vi "XY Graph Delete Successive Plots.vi"(8 "Error In":errorcluster, 9 "Plot Indices":i32[](array[numeric]), 11 "XYGraph Ref":refnum<vi>) -> (0 "Error Out":errorcluster, 1 "Plot Names":string[](array[string]), 2 "Graph Caption":string, 3 "XYGraph Ref":refnum<vi>)   [LabVIEW 2019, in "XY Graph Add-Ons.lvlib"]
uses:
  XY Graph Add-Ons.lvlib
  Plot Update Steps.ctl
  XY Graph Plot Properties.ctl
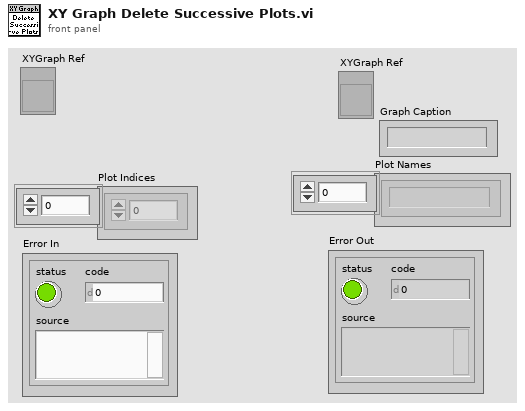
[diagram p1: front panel]
types:
  T1 = typedef "Plot Update Steps.ctl" = enum16{"Update Plot Styles", "Update Annotation List", "Update Cursor List", "Update Plots", "Quit"}
  T2 = typedef "XY Graph Plot Properties.ctl" = cluster{"Plot Index":i32, "Plot.Bar Plot Style":u8, "Plot.DigitalLineStyle":u8, "Plot.TransitionLocation":u8, "Plot.Transition Type":u8, "Plot.Fill To":i16, "Plot.Fill/Pt. Color":u32, "Plot.Label Format":u8, "Plot.Line Style":u8, "Plot.Line Width":u8, "Plot.Plot Color":u32, "Plot.Plot Interpolation":u8, "Plot.Plot Name":string, "Plot.Point Style":u8, "Plot.Visible?":bool, "Plot.XScaleIdx":u32, "Plot.YScaleIdx":u32, "Plot.Anti-aliased":bool}
  T3 = typedef "LVAnnotationListTypeDef.ctl" = cluster{"Name":string, "Color":u32, "Style":u8, "Point Style":u8, "Name Visible":bool, "Allow Drag":bool, "Annotation Mode":u32, "Plot":i32, "Index":i32, "Position":cluster{"X":dbl, "Y":dbl}, "X Scale":u32, "Y Scale":u32, "Show Arrow":bool, "Lock Name":bool, "Plot Area":i32, "Label Offset":cluster{"X":dbl, "Y":dbl}}[]
  T4 = typedef "LVCursorListTypeDef.ctl" = cluster{"Name":string, "Color":u32, "Style":u8, "Point Style":u8, "Name Visible":bool, "Allow Drag":bool, "Cursor Mode":u32, "Plot":i32, "Index":i32, "Position":cluster{"X":dbl, "Y":dbl}, "X Scale":u32, "Y Scale":u32, "Watch Plots":i32[], "Watch All Plots":bool, "Plot Area":i32, "Label Offset":cluster{"X":dbl, "Y":dbl}}[]
  T5 = typedef "XY Graph Add-Ons.lvlib/XY Graph Refnum.ctl" = refnum<vi>
  T6 = cluster{"Name":string, "Color":u32, "Style":u8, "Point Style":u8, "Name Visible":bool, "Allow Drag":bool, "Annotation Mode":u32, "Plot":i32, "Index":i32, "Position":cluster{"X":dbl, "Y":dbl}, "X Scale":u32, "Y Scale":u32, "Show Arrow":bool, "Lock Name":bool, "Plot Area":i32, "Label Offset":cluster{"X":dbl, "Y":dbl}}
  T7 = cluster{"Name":string, "Color":u32, "Style":u8, "Point Style":u8, "Name Visible":bool, "Allow Drag":bool, "Cursor Mode":u32, "Plot":i32, "Index":i32, "Position":cluster{"X":dbl, "Y":dbl}, "X Scale":u32, "Y Scale":u32, "Watch Plots":i32[], "Watch All Plots":bool, "Plot Area":i32, "Label Offset":cluster{"X":dbl, "Y":dbl}}
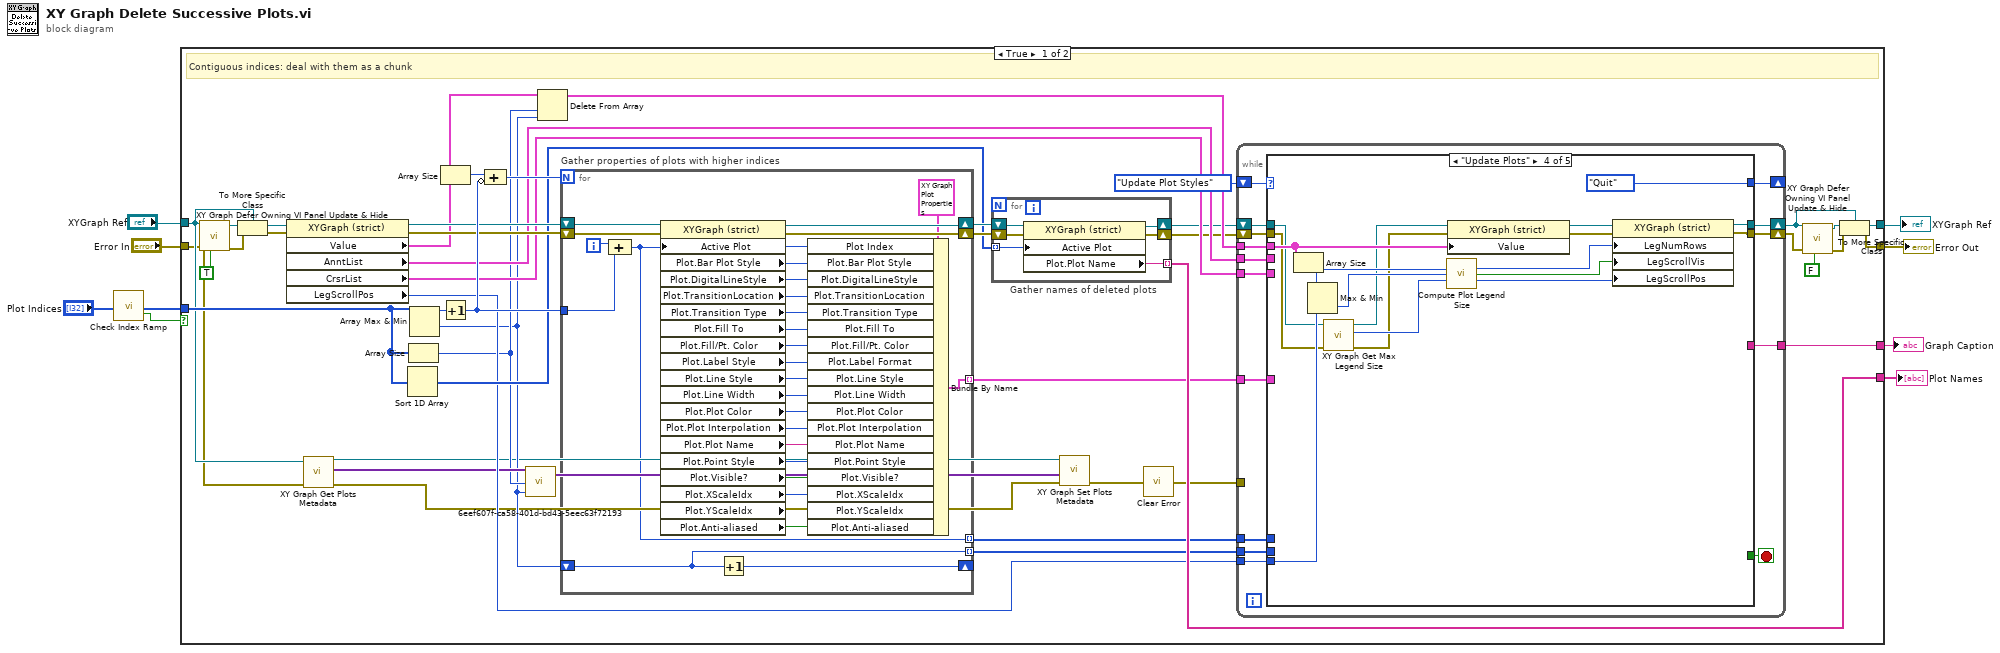
[diagram p0: block diagram]
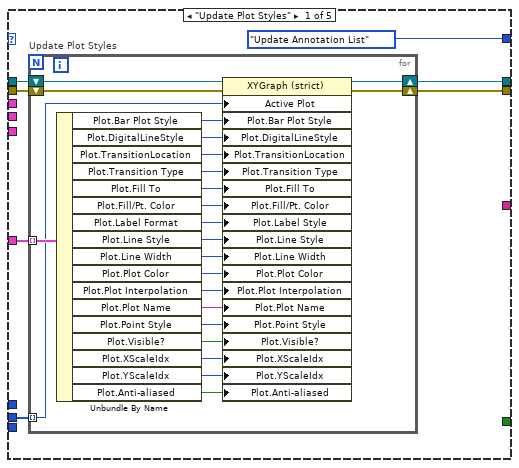
[diagram p2: hidden frame]
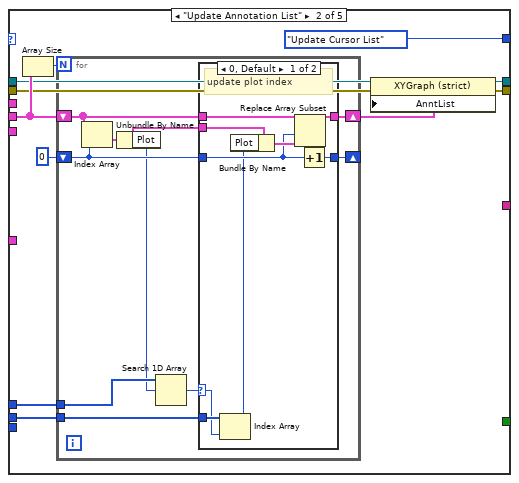
[diagram p3: hidden frame]
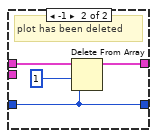
[diagram p4: hidden frame]
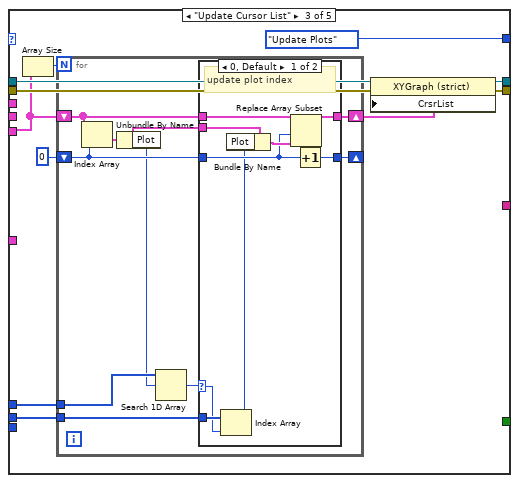
[diagram p5: hidden frame]
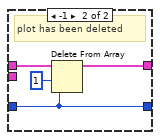
[diagram p6: hidden frame]
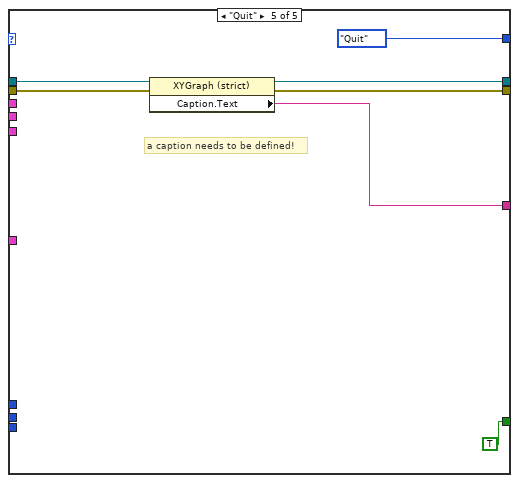
[diagram p7: hidden frame]
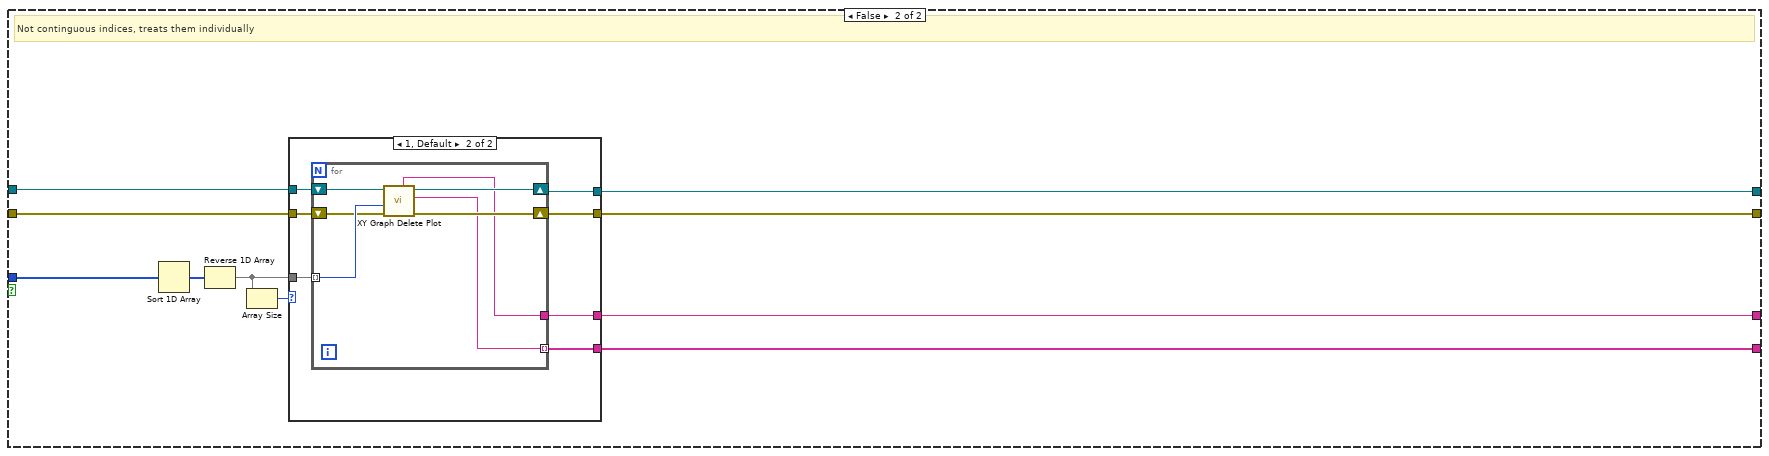
[diagram p8: hidden frame]
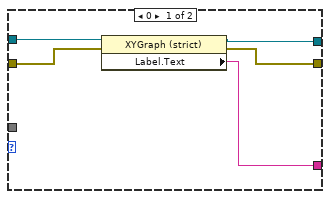
[diagram p9: hidden frame]
diagram:
  n1 = call "Check Index Ramp.vi"("Plot Indices"="Plot Indices") -> ("Plot Indices (dup)"=w1:i32[], "Contiguous?"=w2:bool)  [unwired: 16 in, 1 out]
  n2 = case shown="True" w2 {
    tunnel: "XYGraph Ref" -> [w19 w231]
    tunnel: [w23 w230] -> w8
    tunnel: "Error In" -> [w18 w229]
    tunnel: [w20 w228] -> w6
    tunnel: [w39 w227] -> w5
    tunnel: [w40 w226] -> w4
    tunnel: w1 -> [w46 w233]
    frame True {
      # "Contiguous indices: deal with them as a chunk"
      n3 = call "XY Graph Defer Owning VI Panel Update & Hide.vi"("Defer Owning Panel Update"=TRUE, "error in (no error)"=w18, "XY Graph Refnum in"=w19) -> ("error out"=w24:errorcluster, "XY Graph Refnum out"=w28:refnum<vi>)  [unwired: 7 in]
      n4 = To More Specific Class(target class=w19, reference=w28, error in=w24) -> (specific class reference=w26:refnum<vi>, error out=w25:errorcluster)
      n5 = property class="XYGraph (strict)"(reference=w26, error in=w25) -> (reference out=w49:refnum<vi>, error out=w48:errorcluster, "Value"=w47:cluster{dbl[], dbl[]}[], "AnntList"=w42:T3, "CrsrList"=w41:T4, "LegScrollPos"=w34:u32)
      n6 = call "XY Graph Get Plots Metadata.vi"("Error In"=w18, "XYGraph Refnum"=w19) -> ("Error Out"=w14:errorcluster, "Plots Metadata"=w17:variant[], "XYGraph Refnum"=w10:T5)  [unwired: 6 in, 1 out]
      n7 = Sort 1D Array(array=w46) -> (sorted array=w35:i32[])
      n8 = Array Size(array=w46) -> (size(s)=w16:i32)
      n9 = Array Max & Min(array=w46) -> (max value=w51:i32, min value=w15:i32)  [unwired: 2 out]
      n10 = Array Size(array=w47) -> (size(s)=w54:i32)
      n11 = Increment(x=w51) -> (x+1=w50:i32)
      n12 = Compound Arithmetic op=ADD(w54, invert w50) -> (w52:i32)
      n13 = call "6eef607f-ca58-401d-bd43-5eec63f72193.vi"("index (last elem)"=w15, "length (1)"=w16, "Array"=w17) -> ("array w/ subset deleted"=w11:variant[])  [unwired: 1 out]
      n14 = Delete From Array(array=w47, length=w16, index=w15) -> (array with subset deleted=w45:cluster{dbl[], dbl[]}[])  [unwired: 1 out]
      n15 = for "Gather properties of plots with higher indices" {
        N: w52 -> [_]
        shift-right: [w213] -> w43
        shift-left: w48 -> [w214]
        shift-right: [w215] -> w44
        shift-left: w49 -> [w217]
        tunnel: w50 -> [w195]
        shift-right: [w194] -> _
        shift-left: w15 -> [w193]
        tunnel: [w193] -> w38 mode=indexing
        tunnel: [w192] -> w37 mode=indexing
        tunnel: [w191] -> w36 mode=indexing
        i -> [w216]
        n16 = Compound Arithmetic op=ADD(w216, w195) -> (w191:i32)
        n17 = property class="XYGraph (strict)"(reference=w217, error in=w214, "Active Plot"=w191) -> (reference out=w215:refnum<vi>, error out=w213:errorcluster, "Plot.Bar Plot Style"=w212:u8, "Plot.DigitalLineStyle"=w211:u8, "Plot.TransitionLocation"=w210:u8, "Plot.Transition Type"=w209:u8, "Plot.Fill To"=w208:i16, "Plot.Fill/Pt. Color"=w207:u32, "Plot.Label Style"=w206:u8, "Plot.Line Style"=w205:u8, "Plot.Line Width"=w204:u8, "Plot.Plot Color"=w203:u32, "Plot.Plot Interpolation"=w202:u8, "Plot.Plot Name"=w201:string, "Plot.Point Style"=w200:u8, "Plot.Visible?"=w199:bool, "Plot.XScaleIdx"=w198:u32, "Plot.YScaleIdx"=w197:u32, "Plot.Anti-aliased"=w190:bool)
        n18 = Increment(x=w193) -> (x+1=w194:i32)
        n19 = Bundle By Name(cluster=T2 {"Plot Index"=0, "Plot.Bar Plot Style"=0, "Plot.DigitalLineStyle"=0, "Plot.TransitionLocation"=0, "Plot.Transition Type"=0, "Plot.Fill To"=0, "Plot.Fill/Pt. Color"=0, "Plot.Label Format"=0, "Plot.Line Style"=0, "Plot.Line Width"=0, "Plot.Plot Color"=0, "Plot.Plot Interpolation"=0, "Plot.Plot Name"="", "Plot.Point Style"=0, "Plot.Visible?"=FALSE, "Plot.XScaleIdx"=0, "Plot.YScaleIdx"=0, "Plot.Anti-aliased"=FALSE}, "Plot Index"=w191, "Plot.Bar Plot Style"=w212, "Plot.DigitalLineStyle"=w211, "Plot.TransitionLocation"=w210, "Plot.Transition Type"=w209, "Plot.Fill To"=w208, "Plot.Fill/Pt. Color"=w207, "Plot.Label Format"=w206, "Plot.Line Style"=w205, "Plot.Line Width"=w204, "Plot.Plot Color"=w203, "Plot.Plot Interpolation"=w202, "Plot.Plot Name"=w201, "Plot.Point Style"=w200, "Plot.Visible?"=w199, "Plot.XScaleIdx"=w198, "Plot.YScaleIdx"=w197, "Plot.Anti-aliased"=w190) -> (w192:T2)
      }
      n20 = for "Gather names of deleted plots" {
        shift-right: [w220] -> w32
        shift-left: w43 -> [w221]
        shift-right: [w222] -> w33
        shift-left: w44 -> [w223]
        tunnel: w35 -> [w219] mode=indexing
        tunnel: [w218] -> w40 mode=indexing
        n21 = property class="XYGraph (strict)"(reference=w223, error in=w221, "Active Plot"=w219) -> (reference out=w222:refnum<vi>, error out=w220:errorcluster, "Plot.Plot Name"=w218:string)
      }
      n22 = call "XY Graph Set Plots Metadata.vi"("error in (no error)"=w14, "Plots Metadata"=w11, "XY Graph Refnum"=w10) -> ("error out"=w13:errorcluster)  [unwired: 7 in, 1 out]
      n23 = call "Clear Error.vi"("Error In"=w13) -> ("no Error Out"=w12:errorcluster)  [unwired: 8 in]
      n24 = while {
        shift-right: [w64] -> _
        shift-left: Plot_Update_Steps."Update Plot Styles" -> [w66]
        shift-right: [w60] -> w31
        shift-left: w32 -> [w68]
        tunnel: w42 -> [w63]
        tunnel: w45 -> [w62]
        tunnel: w41 -> [w61]
        shift-right: [w67] -> w22
        shift-left: w33 -> [w69]
        tunnel: [w59] -> w39
        tunnel: w38 -> [w58]
        tunnel: w37 -> [w57]
        tunnel: w36 -> [w56]
        tunnel: w34 -> [w55]
        tunnel: w12 -> [_]
        stop <- w65 stop-if-true
        n25 = case shown="\"Update Plots\"" w66 {
          tunnel: w69 -> [w76 w106 w139 w168 w188]
          tunnel: w68 -> [w75 w104 w137 w169 w185]
          tunnel: [w74 w103 w136 w178 w184] -> w60
          tunnel: [w73 w105 w138 w179 w186] -> w67
          tunnel: w58 -> [w70 w101 w142 _ _]
          tunnel: [_ _ _ _ TRUE] -> w65
          tunnel: [Plot_Update_Steps."Update Annotation List" Plot_Update_Steps."Update Cursor List" Plot_Update_Steps."Update Plots" Plot_Update_Steps."Quit" Plot_Update_Steps."Quit"] -> w64
          tunnel: w63 -> [_ w109 _ _ _]
          tunnel: w62 -> [_ _ _ w181 _]
          tunnel: w61 -> [_ _ w134 _ _]
          tunnel: [_ _ _ _ w183] -> w59
          tunnel: w57 -> [w71 _ _ _ _]
          tunnel: w56 -> [_ w100 w133 _ _]
          tunnel: w55 -> [_ _ _ w175 _]
          frame "Update Plot Styles" {
            n26 = for "Update Plot Styles" {
              tunnel: w71 -> [w99] mode=indexing
              shift-right: [w95] -> w74
              shift-left: w75 -> [w96]
              shift-right: [w97] -> w73
              shift-left: w76 -> [w98]
              tunnel: w70 -> [w78] mode=indexing
              n27 = Unbundle By Name(w99) -> ("Plot.Bar Plot Style"=w94:u8, "Plot.DigitalLineStyle"=w93:u8, "Plot.TransitionLocation"=w92:u8, "Plot.Transition Type"=w91:u8, "Plot.Fill To"=w90:i16, "Plot.Fill/Pt. Color"=w89:u32, "Plot.Label Format"=w88:u8, "Plot.Line Style"=w87:u8, "Plot.Line Width"=w86:u8, "Plot.Plot Color"=w85:u32, "Plot.Plot Interpolation"=w84:u8, "Plot.Plot Name"=w83:string, "Plot.Point Style"=w82:u8, "Plot.Visible?"=w81:bool, "Plot.XScaleIdx"=w80:u32, "Plot.YScaleIdx"=w79:u32, "Plot.Anti-aliased"=w77:bool)
              n28 = property class="XYGraph (strict)"(reference=w98, error in=w96, "Active Plot"=w78, "Plot.Bar Plot Style"=w94, "Plot.DigitalLineStyle"=w93, "Plot.TransitionLocation"=w92, "Plot.Transition Type"=w91, "Plot.Fill To"=w90, "Plot.Fill/Pt. Color"=w89, "Plot.Label Style"=w88, "Plot.Line Style"=w87, "Plot.Line Width"=w86, "Plot.Plot Color"=w85, "Plot.Plot Interpolation"=w84, "Plot.Plot Name"=w83, "Plot.Point Style"=w82, "Plot.Visible?"=w81, "Plot.XScaleIdx"=w80, "Plot.YScaleIdx"=w79, "Plot.Anti-aliased"=w77) -> (reference out=w97:refnum<vi>, error out=w95:errorcluster)
            }
          }
          frame "Update Annotation List" {
            n29 = Array Size(array=w109) -> (size(s)=w108:i32)
            n30 = for {
              N: w108 -> [_]
              shift-right: [w116] -> w102
              shift-left: w109 -> [w118]
              shift-right: [w115] -> _
              shift-left: 0 -> [w117]
              tunnel: w101 -> [w111]
              tunnel: w100 -> [w114]
              n31 = Index Array(array=w118, index=w117) -> (element=w119:T6)
              n32 = Unbundle By Name(w119) -> ("Plot"=w113:i32)
              n33 = Search 1D Array(1D array=w114, element=w113) -> (index of element=w112:i32)  [unwired: 1 in]
              n34 = case shown="0, Default" w112 {
                selector: w112 -> [w121 _]
                tunnel: w119 -> [w128 _]
                tunnel: w118 -> [w126 w132]
                tunnel: w117 -> [w124 w129]
                tunnel: [w123 w130] -> w116
                tunnel: [w127 w129] -> w115
                tunnel: w111 -> [w122 _]
                frame 0, Default {
                  # "update plot index"
                  n35 = Index Array(array=w122, index=w121) -> (element=w120:i32)
                  n36 = Bundle By Name(cluster=w128, "Plot"=w120) -> (w125:T6)
                  n37 = Replace Array Subset(array=w126, new element=w125, index=w124) -> (w123:T3)
                  n38 = Increment(x=w124) -> (x+1=w127:i32)
                }
                frame -1 {
                  # "plot has been deleted"
                  n39 = Delete From Array(array=w132, length=1, index=w129) -> (array with subset deleted=w130:T3)  [unwired: 1 out]
                }
              }
            }
            n40 = property class="XYGraph (strict)"(reference=w106, error in=w104, "AnntList"=w102) -> (reference out=w105:refnum<vi>, error out=w103:errorcluster)
          }
          frame "Update Cursor List" {
            n41 = Array Size(array=w134) -> (size(s)=w141:i32)
            n42 = for {
              N: w141 -> [_]
              tunnel: w142 -> [w144]
              shift-right: [w149] -> w135
              shift-left: w134 -> [w151]
              shift-right: [w148] -> _
              shift-left: 0 -> [w150]
              tunnel: w133 -> [w147]
              n43 = Index Array(array=w151, index=w150) -> (element=w152:T7)
              n44 = Unbundle By Name(w152) -> ("Plot"=w146:i32)
              n45 = Search 1D Array(1D array=w147, element=w146) -> (index of element=w145:i32)  [unwired: 1 in]
              n46 = case shown="0, Default" w145 {
                selector: w145 -> [w154 _]
                tunnel: w152 -> [w161 _]
                tunnel: w151 -> [w159 w165]
                tunnel: w150 -> [w157 w162]
                tunnel: [w156 w163] -> w149
                tunnel: [w160 w162] -> w148
                tunnel: w144 -> [w155 _]
                frame 0, Default {
                  # "update plot index"
                  n47 = Index Array(array=w155, index=w154) -> (element=w153:i32)
                  n48 = Bundle By Name(cluster=w161, "Plot"=w153) -> (w158:T7)
                  n49 = Replace Array Subset(array=w159, new element=w158, index=w157) -> (w156:T4)
                  n50 = Increment(x=w157) -> (x+1=w160:i32)
                }
                frame -1 {
                  # "plot has been deleted"
                  n51 = Delete From Array(array=w165, length=1, index=w162) -> (array with subset deleted=w163:T4)  [unwired: 1 out]
                }
              }
            }
            n52 = property class="XYGraph (strict)"(reference=w139, error in=w137, "CrsrList"=w135) -> (reference out=w138:refnum<vi>, error out=w136:errorcluster)
          }
          frame "Update Plots" {
            n53 = Array Size(array=w181) -> (size(s)=w176:i32)
            n54 = Max & Min(x=w176, y=w175) -> (min(x,y)=w174:u32)  [unwired: 1 out]
            n55 = call "XY Graph Get Max Legend Size.vi"("Error In"=w169, "XYGraph Refnum"=w168) -> ("Error Out"=w166:errorcluster, "Max Legend Size"=w170:i32, "XYGraph Refnum"=w167:T5)  [unwired: 6 in, 1 out]
            n56 = call "Compute Plot Legend Size.vi"("# Plots"=w176, "Current Plot (Last)"=w174, "Max Legend Size"=w170) -> ("LegNumRows"=w173:u32, "LegScrollVis"=w172:bool, "LegScrollPos"=w171:u32)  [unwired: 10 in]
            n57 = property class="XYGraph (strict)"(reference=w167, error in=w166, "Value"=w181) -> (reference out=w180:T5, error out=w177:errorcluster)
            n58 = property class="XYGraph (strict)"(reference=w180, error in=w177, "LegNumRows"=w173, "LegScrollVis"=w172, "LegScrollPos"=w171) -> (reference out=w179:T5, error out=w178:errorcluster)
          }
          frame "Quit" {
            # "a caption needs to be defined!"
            n59 = property class="XYGraph (strict)"(reference=w188, error in=w185) -> (reference out=w186:refnum<vi>, error out=w184:errorcluster, "Caption.Text"=w183:string)
          }
        }
      }
      n60 = call "XY Graph Defer Owning VI Panel Update & Hide.vi"("Defer Owning Panel Update"=FALSE, "error in (no error)"=w31, "XY Graph Refnum in"=w22) -> ("error out"=w21:errorcluster, "XY Graph Refnum out"=w30:refnum<vi>)  [unwired: 7 in]
      n61 = To More Specific Class(target class=w22, reference=w30, error in=w21) -> (specific class reference=w23:refnum<vi>, error out=w20:errorcluster)
    }
    frame False {
      # "Not continguous indices, treats them individually"
      n62 = Sort 1D Array(array=w233) -> (sorted array=w232:i32[])
      n63 = Reverse 1D Array(array=w232) -> (reversed array=w225:i32[])
      n64 = Array Size(array=w225) -> (size(s)=w224:i32)
      n65 = case shown="1, Default" w224 {
        tunnel: w231 -> [w238 w245]
        tunnel: [w236 w244] -> w230
        tunnel: w229 -> [w237 w243]
        tunnel: [w235 w242] -> w228
        tunnel: [w234 w241] -> w227
        tunnel: [_ w240] -> w226
        tunnel: w225 -> [_ w239]
        frame 0 {
          n66 = property class="XYGraph (strict)"(reference=w238, error in=w237) -> (reference out=w236:refnum<vi>, error out=w235:errorcluster, "Label.Text"=w234:string)
        }
        frame 1, Default {
          n67 = for {
            tunnel: w239 -> [w251] mode=indexing
            shift-right: [w248] -> w242
            shift-left: w243 -> [w249]
            tunnel: [w247] -> w241
            tunnel: [w246] -> w240 mode=indexing
            shift-right: [w250] -> w244
            shift-left: w245 -> [w252]
            n68 = call "XY Graph Delete Plot.vi"("Error In"=w249, "Plot Index"=w251, "XYGraph Ref"=w252) -> ("Error Out"=w248:errorcluster, "Plot Name"=w246:string, "XYGraph Ref"=w250:T5, "Graph Caption (or Label)"=w247:string)  [unwired: 5 in]
          }
        }
      }
    }
  }
  "XYGraph Ref" <- w8
  "Error Out" <- w6
  "Graph Caption" <- w5
  "Plot Names" <- w4
